vi "ble_connection.vi"() -> ()   [LabVIEW 2021]
uses:
  <vilib>/BLE/type_def/address_type.ctl
panel:
  out "payload":u8[](array[numeric])
  out "Handle table":string[][](array[string])
  out "attribute value":u8[](array[numeric])
  in  "COM Bluegiga in":refnum<visa-resource-name>
  out "Bluetooth Status":bool
  in  "stop":bool
  in  "Tab Control":enum32{"Calibration", "Working Page"}(tab)
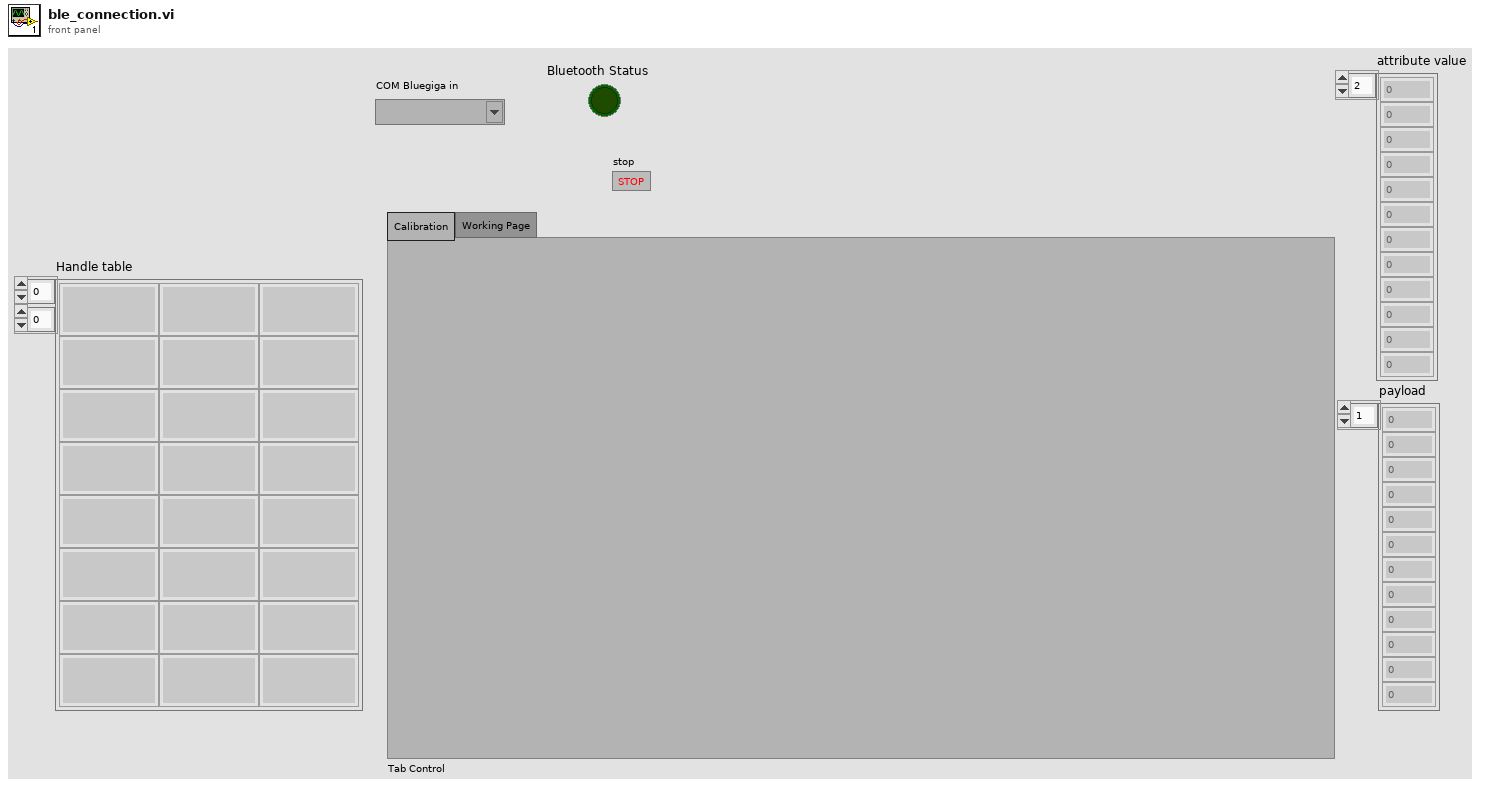
[diagram p1: front panel]
types:
  T1 = typedef "address_type.ctl" = u8
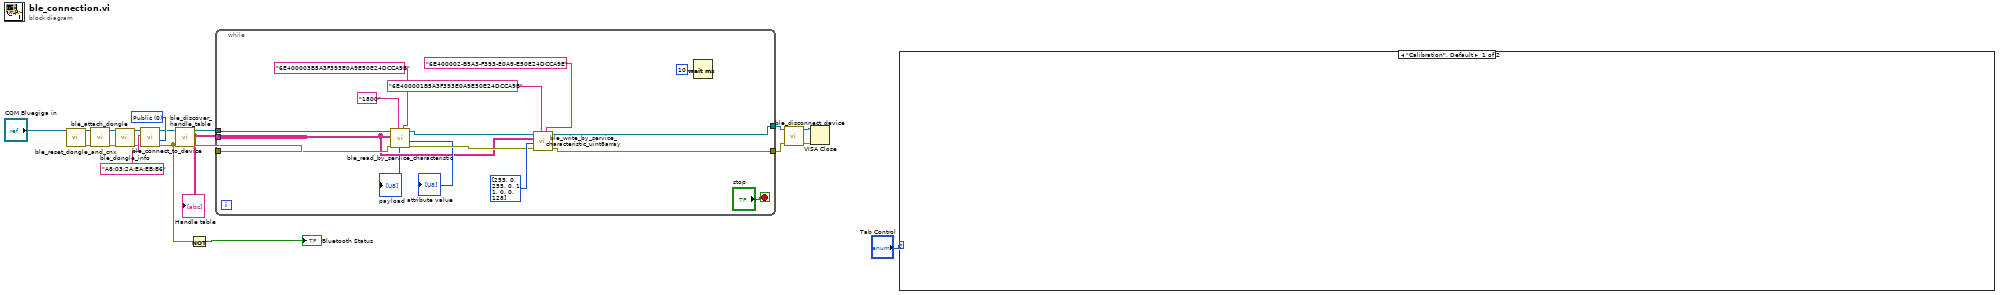
[diagram p0: block diagram]
diagram:
  w12 = T1 0 items=["Public", "Random"] ("Address Type")
  n1 = call <vilib>:"ble_reset_dongle_and_cnx.vi"("COM Bluegiga in"="COM Bluegiga in") -> ("error out"=w17:errorcluster, "COM Bluegiga out"=w16:refnum<visa-resource-name>)  [unwired: 9 in]
  n2 = call <vilib>:"ble_attach_dongle.vi"("error in (no error)"=w17, "COM Bluegiga in"=w16) -> ("error out"=w19:errorcluster, "COM Bluegiga out"=w18:refnum<visa-resource-name>)  [unwired: 8 in]
  n3 = call <vilib>:"ble_dongle_info.vi"("error in (no error)"=w19, "COM Bluegiga in"=w18) -> ("error out"=w13:errorcluster, "COM Bluegiga out"=w14:refnum<visa-resource-name>)  [unwired: 7 in, 1 out]
  n4 = call <vilib>:"ble_connect_to_device.vi"("Address Type"=w12, "error in (no error)"=w13, "MAC Address"="A8:03:2A:EA:EB:B6", "COM Bluegiga in"=w14) -> ("error out"=w5:errorcluster, "COM Bluegiga out"=w6:refnum<visa-resource-name>)  [unwired: 5 in, 1 out]
  n5 = call <vilib>:"ble_discover_handle_table.vi"("error in (no error)"=w5, "COM Bluegiga in"=w6) -> ("error out"=w4:errorcluster, "Handle table"=w3:string[][], "COM Bluegiga out"=w2:refnum<visa-resource-name>)  [unwired: 7 in]
  "Handle table" <- w3
  n6 = Not(x=w5) -> (.not. x?=→"Bluetooth Status":bool)
  n7 = while {
    tunnel: w4 -> [w31]
    tunnel: [w34] -> w9
    tunnel: w2 -> [w32]
    tunnel: [w35] -> w10
    tunnel: w3 -> [w24]
    stop <- "stop" stop-if-true
    n8 = call <vilib>:"ble_read_by_service_characteristic.vi"("Characteristic UUID"="6E400003B5A3F393E0A9E50E24DCCA9E" ("Service UUID"), "Service UUID"="1800", "error in (no error)"=w31, "Handle table"=w24, "COM Bluegiga in"=w32) -> ("error out"=w26:errorcluster, "attribute value"=→"attribute value":u8[], "payload"=→"payload":u8[], "COM Bluegiga out"=w27:refnum<visa-resource-name>)  [unwired: 3 in]
    n9 = call <vilib>:"ble_write_by_service_characteristic_uint8array.vi"("Characteristic UUID"="6E400002-B5A3-F393-E0A9-E50E24DCCA9E" ("Service UUID"), "Service UUID"="6E400001B5A3F393E0A9E50E24DCCA9E", "error in (no error)"=w26, "data"=u8[] [255, 0, 255, 0, 1, 1, 0, 0, 128], "Handle table"=w24, "COM Bluegiga in"=w27) -> ("error out"=w34:errorcluster, "COM Bluegiga out"=w35:refnum<visa-resource-name>)  [unwired: 4 in]
    n10 = Wait (ms)(milliseconds to wait=u32 10) -> ()  [unwired: 1 out]
  }
  n11 = call <vilib>:"ble_disconnect_device.vi"("error in (no error)"=w9, "COM Bluegiga in"=w10) -> ("error out"=w7:errorcluster, "COM Bluegiga out"=w8:refnum<visa-resource-name>)  [unwired: 8 in]
  n12 = VISA Close(VISA resource name=w8, error in (no error)=w7) -> ()  [unwired: 1 out]
  n13 = case shown="\"Calibration\", Default" "Tab Control" {
    frame "Calibration", Default {
    }
    frame "Working Page" {
    }
  }
